vi "USRP Dummy DMA Zero Copy (Host).vi"() -> ()   [LabVIEW 2016]
uses:
  <vilib>/userdefined/High Color/nirio_resource_hc.ctl
  <vilib>/FPGAPlugInAG/USRP 294xR; 295xR 200 MSps/niLvFpga_Open_USRP 294xR; 295xR 200 MSps.vi
  <vilib>/rvi/interface/common/dynamic/niFpgaDynamicAddResources.vi
  <vilib>/FPGAPlugInAG/Dynamic/niLvFpga_Download_Dynamic.vi
  <vilib>/FPGAPlugInAG/Dynamic/niLvFpga_Run_Dynamic.vi
  <vilib>/Utility/error.llb/Error Cluster From Error Code.vi
  <vilib>/rvi/errors/niLvFpgaAdjustHostInterfaceError.vi
  <vilib>/rvi/interface/common/niFpgaWaitOnOcc.vi
  <vilib>/FPGAPlugInAG/Dynamic/niLvFpga_Close_Dynamic.vi
  <vilib>/rvi/interface/nirviOpenFPGA/nirviOpenFPGA.xnode
  FPGA Bitfiles/USRP-RIO-Streami_DummyDMA_USRPDummyv2(FPGA_kYza4iCu9yA.lvbitx
  <vilib>/rvi/interface/nirviMethod/nirviMethod.xnode
  <vilib>/rvi/interface/nirviReadWriteControl/nirviReadWriteControl.xnode
  <vilib>/rvi/interface/nirviCloseFPGA/nirviCloseFPGA.xnode
  <vilib>/rvi/errors/niLvFpgaMergeErrorWithErrorCode.vi
  <vilib>/rvi/interface/Simulation/niFpgaSimulationCallBeginRW.vi
  <instrlib>/niUsrpRio/Config/v1/Host/niUsrpRio Config v1 Host.lvlib
  NiFpgaLv.dll
  <vilib>/FPGAPlugInAG/Dynamic/niLvFpga_StopFifo_Dynamic.vi
  <vilib>/FPGAPlugInAG/Dynamic/niLvFpga_ConfigureFifo_Dynamic.vi
  <vilib>/FPGAPlugInAG/Dynamic/niLvFpga_StartFifo_Dynamic.vi
  <vilib>/FPGAPlugInAG/Dynamic/niLvFpga_AcquireReadRegionFifo_Dynamic.vi
panel:
  out "Random Generator":u8
  in  "Decimate (200 MHz)":u32=5
  in  "file path":path=path "C:/Users/jfernand/Desktop/USRP-RIO-Streaming/Streams/Dummy-DMA-TDMS-Test-File.tdms"
  out "Host Transfer Slider":u64(slide) scale=0.0..1073741824.0
  in  "Flush FIFO?":bool
  out "Control Loop":i32
  in  "Host FIFO Fetch":u64=131072
  in  "Reset Host Count?":bool
  in  "Stop Transfer?":bool
  in  "Reset FPGA Count?":bool
  out "FPGA Side FIFO":cluster{u32, u32}(slide)={66, 63} scale=0.0..2047.0
  out "Host TDMS Buffer":cluster{u32, u32}(slide) scale=0.0..67108863.0
  out "Data Loop":i32
  out "Fetch Loop":i32
  out "Host Count":u64
  in  "Number of Samples":u64=1073741824
  out "FPGA Count":u64
  in  "Start Transfer":bool
  in  "Terminate":bool
  out "Elements Remaining":u32
  out "Data":u64[](array[numeric]) format="%016x"
  out "Timeout Counts":u64
  in  "Reset Timeouts?":bool
  out "Actual Depth":u32
  in  "Host Requested Depth":u32=67108864
  out "error out":errorcluster
  in  "error in (no error)":errorcluster
  in  "resource name":T1="PXI2Slot18Port1Dev1"
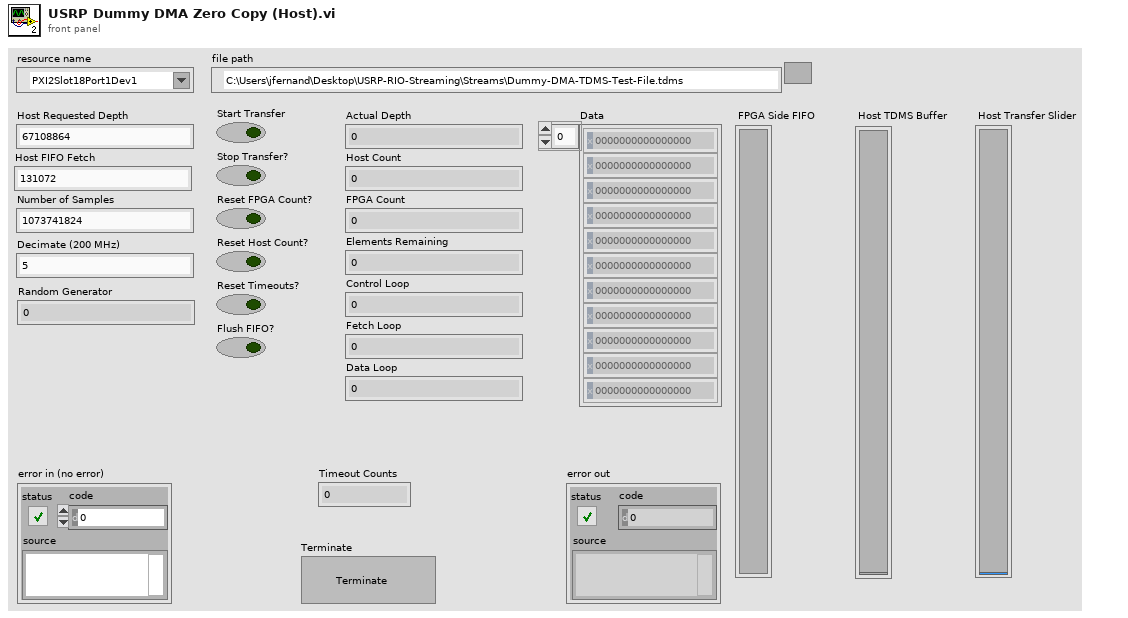
[diagram p1: front panel]
types:
  T1 = typedef "nirio_resource_hc.ctl" = tag
  T2 = enum16{"open", "open or create", "create or replace", "create", "open (read-only)"}
  T3 = typedef "niUsrpRio Config v1 Host.lvlib/niUsrpRio Session.ctl" = cluster{"FPGA Interface":refnum<k20>, "RIO Interface Number":u32, "Data Clock Rate":u32, "FPGA Data Clock Rate":u32, "Global Settings Register Bus":T4, "Radio 0 Settings Register Bus":T4, "Radio 1 Settings Register Bus":T4, "Radio Settings Bus Semaphore":T5, "DB Queues":T6[], "Characterization Data Valid?":bool, "EEPROM Header":T7, "Device Data Header":T8, "EEPROM Characterization Header":T9, "Characterization Data":T10[], "FPGA Current Version":u32, "FPGA Oldest Compatible Version":u32, "Fixed Logic Current Version":u32, "Fixed Logic Oldest Compatible Version":u32, "FPGA Radio Settings Bus Current Version":u32, "FPGA Radio Settings Bus Oldest Compatible Version":u32, "FPGA Board Config Current Version":u32, "FPGA Board Config Oldest Compatible Version":u32, "Daughterboard Clock Rate":u32, "daughterboard configuration session handles":u64[]}
  T4 = typedef "niInstr Register Bus v0 Host.lvlib/Register Bus Session.ctl" = refnum<queue>
  T5 = typedef "Semaphore RefNum" = refnum<k1>
  T6 = typedef "niUsrpRio Config v1 Host.lvlib/DB Queue Reference.ctl" = refnum<queue>
  T7 = typedef "niUsrpRio Config v1 Host.lvlib/EEPROM Header.ctl" = cluster{"Checksum":u32, "Product Code":u16, "Hardware Current Version":u16, "Hardware Oldest Compatible Version":u16, "EEPROM Map Current Version":u16, "EEPROM Map Oldest Compatible Version":u16, "User Password":string, "Pointer to Factory Header":u32, "Pointer to User Header":u32, "Recommended Interval":u16, "Number of Reserved Bytes":i32, "Number of Daughterboards":u8, "Daughterboard IDs":u16[], "Daughterboard Serial Numbers":string[]}
  T8 = typedef "niUsrpRio Config v1 Host.lvlib/EEPROM Device Data Header.ctl" = cluster{"Checksum":u32, "Number of Channels":u8, "Number of Gain Settings":u16[], "Pointer to Characterization Data":u32[], "Number of Reserved Bytes":i32, "Number of Frequencies":u16[]}
  T9 = typedef "niUsrpRio Config v1 Host.lvlib/EEPROM Characterization Header.ctl" = cluster{"Checksum":u32, "Date":timestamp, "Temperature":sgl, "Misc. Info":string, "Pointer to Device Data Header":u32, "Number of Reserved Bytes":i32}
  T10 = typedef "niUsrpRio Config v1 Host.lvlib/Characterization Data.ctl" = cluster{"Gains[dB]":dbl[], "Frequencies [Hz]":dbl[], "IQ Imbalance Table":T11[], "Measured Gains[dB]":dbl[][]}
  T11 = typedef "niUsrpRio Config v1 Host.lvlib/IQ Imbalance.ctl" = cluster{"Gain Imbalance [linear]":dbl, "Phase Imbalance [radians]":dbl, "Offset":cdb}
  T12 = cluster{"Running Max":u32, "Elements Remaining":u32}
  T13 = cluster{"Maximum Amount Used":u32, "Current Amount Used":u32}
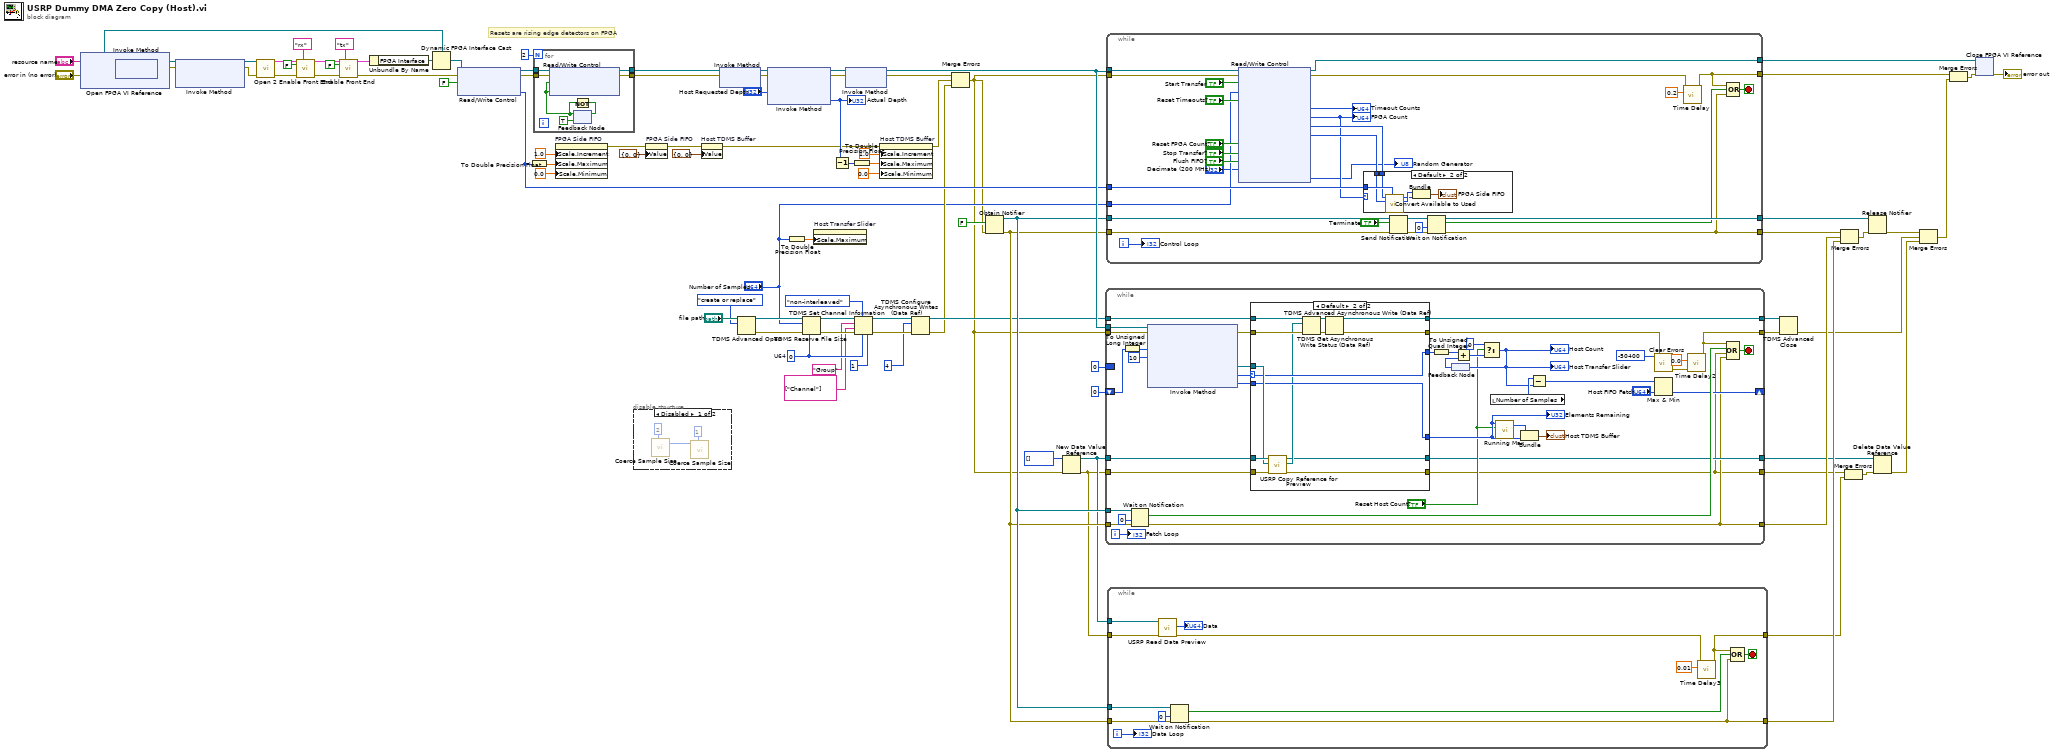
[diagram p0: block diagram]
diagram:
  w23 = u64 0  # U64
  # "Resets are rising edge detectors on FPGA"
  n1 = xnode "Open FPGA VI Reference"("error in"="error in (no error)", "resource name"="resource name") -> ("FPGA VI Reference Out"=w36:refnum<k20>, "error out"=w35:errorcluster)
  n2 = xnode "Invoke Method"("FPGA VI Reference In"=w36, "error in"=w35) -> ("FPGA VI Reference Out"=w34:refnum<k20>, "error out"=w33:errorcluster)
  n3 = xnode "Invoke Method"("FPGA VI Reference In"=w34, "error in"=w33) -> ("FPGA VI Reference Out"=w32:refnum<k20>, "error out"=w31:errorcluster)  [unwired: 1 in]
  n4 = call <instrlib>:"Open 2.vi"("fpga ref"=w32, "error in"=w31) -> ("niUsrpRio Session (out)"=w83:T3, "error out"=w88:errorcluster)  [unwired: 12 in]
  n5 = call <instrlib>:"Enable Front End.vi"("niUsrpRio Session"=w83, "scope"="rx", "enable"=FALSE, "error in"=w88) -> ("niUsrpRio Session (out)"=w84:T3, "error out"=w87:errorcluster)  [unwired: 10 in]
  n6 = call <instrlib>:"Enable Front End.vi"("niUsrpRio Session"=w84, "scope"="tx", "enable"=FALSE, "error in"=w87) -> ("niUsrpRio Session (out)"=w80:T3, "error out"=w79:errorcluster)  [unwired: 10 in]
  n7 = Unbundle By Name(w80) -> ("FPGA Interface"=w78:refnum<k20>)
  n8 = Dynamic FPGA Interface Cast(Session In=w36, Type=w78) -> (Session Out=w77:refnum<k20>)
  n9 = xnode "Read/Write Control"("FPGA VI Reference In"=w77, "error in"=w79, "Start Transfer?"=FALSE ("send data?")) -> ("FPGA VI Reference Out"=w62:refnum<k20>, "error out"=w61:errorcluster, "FPGA FIFO Depth"=w48:u32)
  n10 = To Double Precision Float(number=w48) -> (double precision float=w50:dbl)
  n11 = for {
    N: 2 -> [_]
    tunnel: w62 -> [w101]
    tunnel: w61 -> [w100]
    tunnel: [w99] -> w60
    tunnel: [w98] -> w59
    n12 = feedback #1(TRUE) -> (w96:bool)
    n13 = xnode "Read/Write Control"("FPGA VI Reference In"=w101, "error in"=w100, "Reset Timeouts?"=w96, "Reset FPGA Count?"=w96) -> ("FPGA VI Reference Out"=w99:refnum<k20>, "error out"=w98:errorcluster)
    n14 = Not(x=w96) -> (.not. x?=w95:bool)
    n15 = feedback-in #1(w95) -> ()
  }
  n16 = property on="FPGA Side FIFO" class="Slide (strict)"("Scale.Increment"=1.0 ("Scale.Range:Increment"), "Scale.Maximum"=w50, "Scale.Minimum"=0.0 ("Scale.Range:Minimum")) -> (error out=w43:errorcluster)  [unwired: 2 in, 1 out]
  n17 = disable-structure shown="Disabled" {
    frame Disabled {
      n18 = call "Coerce Sample Size.vi"("Bytes Per Sample (B)"=u64 2) -> ("Coerced Size (samples)"=w104:u64)  [unwired: 6 in]
      n19 = call "Coerce Sample Size.vi"("Bytes Per Sample (B)"=u64 1, "Size (samples)"=w104) -> ()  [unwired: 5 in, 1 out]
    }
    frame Enabled {
    }
  }
  n20 = property on="FPGA Side FIFO" class="Slide (strict)"(error in=w43, "Value"=cluster{u32, u32} {0, 0} ("FPGA Side FIFO")) -> (error out=w46:errorcluster)  [unwired: 1 in, 1 out]
  n21 = property on="Host TDMS Buffer" class="Slide (strict)"(error in=w46, "Value"=cluster{u32, u32} {0, 0} ("FPGA Side FIFO")) -> (error out=w42:errorcluster)  [unwired: 1 in, 1 out]
  n22 = xnode "Invoke Method"("FPGA VI Reference In"=w60, "error in"=w59) -> ("FPGA VI Reference Out"=w94:refnum<k20>, "error out"=w93:errorcluster)
  n23 = TDMS Advanced Open(10:T2."create or replace" ("operation (0:open)"), 11:"file path") -> (0:w26:errorcluster, 3:w27:refnum<k34>)  [unwired: 3 in, 1 out]
  n24 = xnode "Invoke Method"("FPGA VI Reference In"=w94, "error in"=w93, "Requested Depth"="Host Requested Depth") -> ("FPGA VI Reference Out"=w90:refnum<k20>, "error out"=w91:errorcluster, "Actual Depth"=w47:u32)
  "Actual Depth" <- w47
  n25 = To Double Precision Float(number="Number of Samples") -> (double precision float=w10:dbl)
  n26 = TDMS Reserve File Size(6:w23, 8:w26, 10:"Number of Samples", 11:w27) -> (0:w24:errorcluster, 3:w25:refnum<k34>)  [unwired: 1 in]
  n27 = property on="Host Transfer Slider" class="Slide (strict)"("Scale.Maximum"=w10) -> ()  [unwired: 2 in, 2 out]
  n28 = Decrement(x=w47) -> (x-1=w53:u32)
  n29 = xnode "Invoke Method"("FPGA VI Reference In"=w90, "error in"=w91) -> ("FPGA VI Reference Out"=w74:refnum<k20>, "error out"=w49:errorcluster)
  n30 = To Double Precision Float(number=w53) -> (double precision float=w37:dbl)
  n31 = TDMS Set Channel Information(4:u32 1 ("samples per channel"), 6:w23, 7:enum16{"non-interleaved", "interleaved"}."non-interleaved" ("data layout (0:non-interleaved)"), 8:w24, 9:string[] ["Channel"] ("channel name(s)"), 10:"Group" ("group name (Untitled)"), 11:w25) -> (0:w19:errorcluster, 3:w20:refnum<k34>)
  n32 = property on="Host TDMS Buffer" class="Slide (strict)"(error in=w42, "Scale.Increment"=1.0 ("Data Entry Limits:Increment"), "Scale.Maximum"=w37, "Scale.Minimum"=0.0 ("Data Entry Limits:Minimum")) -> (error out=w41:errorcluster)  [unwired: 1 in, 1 out]
  n33 = TDMS Configure Asynchronous Writes (Data Ref)(8:w19, 10:u32 4 ("max asynchronous writes (4)"), 11:w20) -> (0:w14:errorcluster, 3:w15:refnum<k34>)  [unwired: 1 in]
  n34 = Merge Errors(w49, w41, w14) -> (w6:errorcluster)
  n35 = Obtain Notifier(notification data type=FALSE, error in (no error)=w6) -> (notifier out=w66:refnum<notifier>, error out=w65:errorcluster)  [unwired: 2 in, 1 out]
  n36 = New Data Value Reference(data value=u64[] [] ("Data"), error in=w6) -> (data value reference=w7:refnum<data-value>, error out=w4:errorcluster)
  n37 = while {
    tunnel: [w140] -> w13
    tunnel: w74 -> [w143]
    tunnel: w6 -> [w142]
    border: u64 0 -> [_]
    tunnel: w66 -> [w136]
    tunnel: w65 -> [w135]
    tunnel: [w106] -> w68
    tunnel: w4 -> [w132]
    tunnel: [w105] -> w3
    shift-right: [w125] -> _
    shift-left: u64 0 -> [w126]
    tunnel: w15 -> [w118]
    tunnel: [w117] -> w12
    tunnel: w7 -> [w114]
    tunnel: [w107] -> w5
    i -> [w133]
    stop <- w138 stop-if-true
    n38 = To Unsigned Long Integer(number=w126) -> (unsigned 32bit integer=w124:u32)
    n39 = Wait on Notification(notifier=w136, timeout in ms (-1)=0, error in (no error)=w135) -> (notification=w134:bool, error out=w106:errorcluster)  [unwired: 1 in, 2 out]
    n40 = xnode "Invoke Method"("FPGA VI Reference In"=w143, "error in"=w142, "Number of Elements"=w124, "Timeout (ms)"=10) -> ("error out"=w120:errorcluster, "Read Region Reference"=w115:refnum<data-value>, "Elements In Region"=w116:u32, "Elements Remaining"=w113:u32)  [unwired: 1 out]
    n41 = case shown="Default" w116 {
      selector: w116 -> [w147 w154]
      tunnel: w132 -> [w149 w165]
      tunnel: [w149 w164] -> w105
      tunnel: w120 -> [w150 w163]
      tunnel: [w150 w162] -> w119
      tunnel: w113 -> [w148 w155]
      tunnel: w118 -> [w151 w161]
      tunnel: [w151 w160] -> w117
      tunnel: w115 -> [_ w156]
      tunnel: w114 -> [w146 w157]
      tunnel: [w148 w155] -> w109
      tunnel: [w147 w154] -> w112
      tunnel: [w146 w152] -> w107
      frame 0 {
      }
      frame Default {
        n42 = call "USRP Copy Reference for Preview.vi"("error in (no error)"=w165, "FPGA FIFO Reference in"=w156, "Data Preview Reference in"=w157) -> ("error out"=w164:errorcluster, "FPGA FIFO Reference out"=w153:refnum<data-value>, "Data Preview Reference out"=w152:refnum<data-value>)  [unwired: 6 in]
        n43 = TDMS Advanced Asynchronous Write (Data Ref)(8:w163, 10:w153, 11:w161) -> (0:w158:errorcluster, 3:w159:refnum<k34>)  [unwired: 1 in]
        n44 = TDMS Get Asynchronous Write Status (Data Ref)(8:w158, 11:w159) -> (0:w162:errorcluster, 3:w160:refnum<k34>)  [unwired: 1 out]
      }
    }
    "Elements Remaining" <- w109
    n45 = To Unsigned Quad Integer(1:w112) -> (0:w145:u64)
    n46 = feedback #2() -> (w144:u64)
    n47 = Add(x=w145, y=w144) -> (x+y=w131:u64)
    n48 = Select(t=u64 0, s="Reset Host Count?", f=w131) -> (s? t:f=w128:u64)
    "Host Count" <- w128
    "Host Transfer Slider" <- w128
    n49 = feedback-in #2(w128) -> ()
    n50 = local read "Number of Samples"() -> (w129:u64)
    n51 = call "Running Max.vi"("Reset"="Reset Host Count?", "Next Value"=w109) -> ("Running Max"=w111:u32)  [unwired: 5 in]
    n52 = Bundle("Running Max"=w111, "Elements Remaining"=w109) -> (→"Host TDMS Buffer":T12)  [unwired: 1 in]
    n53 = Subtract(x=w129, y=w128) -> (x-y=w127:u64)
    n54 = call <vilib>:"Clear Errors.vi"("error in (no error)"=w119, "specific error code to clear (0: all)"=-50400) -> ("error out"=w123:errorcluster)  [unwired: 4 in, 1 out]
    n55 = Max & Min(x=w127, y="Host FIFO Fetch") -> (min(x,y)=w125:u64)  [unwired: 1 out]
    n56 = call "Time Delay2"("error in (no error)"=w123, "Delay Time (s)"=0.0) -> ("error out"=w140:errorcluster)  [unwired: 9 in]
    n57 = Compound Arithmetic op=OR(w140, w134, w105, w106) -> (w138:bool)
    "Fetch Loop" <- w133
  }
  n58 = while {
    tunnel: w74 -> [w195]
    tunnel: w6 -> [w194]
    tunnel: w66 -> [w191]
    tunnel: w65 -> [w190]
    tunnel: [w185] -> w71
    tunnel: [w178] -> w70
    tunnel: [w180] -> w58
    tunnel: [w179] -> w57
    tunnel: w48 -> [w177]
    tunnel: "Number of Samples" -> [w168]
    i -> [w170]
    stop <- w184 stop-if-true
    n59 = xnode "Read/Write Control"("FPGA VI Reference In"=w195, "error in"=w194, "Start Transfer?"="Start Transfer", "Number of Samples"=w168, "Reset Timeouts?"="Reset Timeouts?", "Reset Timeouts?"="Reset FPGA Count?", "Stop Transfer?"="Stop Transfer?", "Flush FIFO?"="Flush FIFO?", "Decimate (200MHz)"="Decimate (200 MHz)") -> ("FPGA VI Reference Out"=w179:refnum<k20>, "error out"=w193:errorcluster, "Timeout Count"=→"Timeout Counts":u64, "FPGA Count"=w171:u64, "Space Available"=w176:u32, "Min Space Available"=w174:u32, "Random Number"=→"Random Generator":u8)
    "FPGA Count" <- w171
    n60 = case shown="Default" w171 {
      tunnel: w177 -> [_ w201]
      tunnel: w176 -> [_ w200]
      tunnel: w174 -> [_ w199]
      frame 0 {
      }
      frame Default {
        n61 = call "Convert Available to Used.vi"("Size"=w201, "Minimum Amount Available"=w199, "Current Amount Available"=w200) -> ("Maximum Amount Used"=w198:u32, "Current Amount Used"=w197:u32)  [unwired: 5 in]
        n62 = Bundle("Maximum Amount Used"=w198, "Current Amount Used"=w197) -> (→"FPGA Side FIFO":T13)  [unwired: 1 in]
      }
    }
    n63 = Send Notification(notification="Terminate", notifier=w191, error in (no error)=w190) -> (notifier out=w187:refnum<notifier>, error out=w186:errorcluster)
    n64 = Wait on Notification(notifier=w187, timeout in ms (-1)=0, error in (no error)=w186) -> (notifier out=w185:refnum<notifier>, notification=w183:bool, error out=w178:errorcluster)  [unwired: 1 in, 1 out]
    n65 = call "Time Delay"("error in (no error)"=w193, "Delay Time (s)"=0.2) -> ("error out"=w180:errorcluster)  [unwired: 9 in]
    n66 = Compound Arithmetic op=OR(w180, w183, w178) -> (w184:bool)
    "Control Loop" <- w170
  }
  n67 = while {
    tunnel: w66 -> [w212]
    tunnel: w65 -> [w211]
    tunnel: [w206] -> w64
    tunnel: w7 -> [w205]
    tunnel: [w208] -> w63
    tunnel: w4 -> [w203]
    i -> [w214]
    stop <- w209 stop-if-true
    n68 = call "USRP Read Data Preview.vi"("error in (no error)"=w203, "Data Value Reference in"=w205) -> ("error out"=w202:errorcluster, "Data"=→"Data":u64[])  [unwired: 7 in, 1 out]
    n69 = Wait on Notification(notifier=w212, timeout in ms (-1)=0, error in (no error)=w211) -> (notification=w210:bool, error out=w206:errorcluster)  [unwired: 1 in, 2 out]
    n70 = call "Time Delay3"("error in (no error)"=w202, "Delay Time (s)"=0.01) -> ("error out"=w208:errorcluster)  [unwired: 9 in]
    n71 = Compound Arithmetic op=OR(w208, w210, w206) -> (w209:bool)
    "Data Loop" <- w214
  }
  n72 = TDMS Advanced Close(8:w13, 11:w12) -> (0:w11:errorcluster)  [unwired: 2 in, 1 out]
  n73 = Merge Errors(w70, w68, w64) -> (w69:errorcluster)
  n74 = Merge Errors(w3, w63) -> (w2:errorcluster)
  n75 = Release Notifier(notifier=w71, error in (no error)=w69) -> (error out=w67:errorcluster)  [unwired: 1 in, 2 out]
  n76 = Delete Data Value Reference(data value reference=w5, error in=w2) -> (error out=w1:errorcluster)  [unwired: 1 out]
  n77 = Merge Errors(w67, w11, w1) -> (w38:errorcluster)
  n78 = Merge Errors(w58, w38) -> (w39:errorcluster)
  n79 = xnode "Close FPGA VI Reference"("FPGA VI Reference In"=w57, "error in"=w39) -> ("error out"=→"error out":errorcluster)
